vi "Deinit.vi"(8 "error in (no error)":errorcluster, 11 "AcquistionObject in":refnum<class "AcquistionObject.lvclass">) -> (0 "error out":errorcluster, 3 "AcquistionObject out":refnum<class "AcquistionObject.lvclass">)   [LabVIEW 2014, in "AcquisitionCoreObjects.lvlib" / "AcquistionObject.lvclass"]
uses:
  AcquistionObject.lvclass
  <vilib>/Utility/config.llb/NI_LVConfig.lvlib
  <vilib>/addons/database/NI_Database_API.lvlib
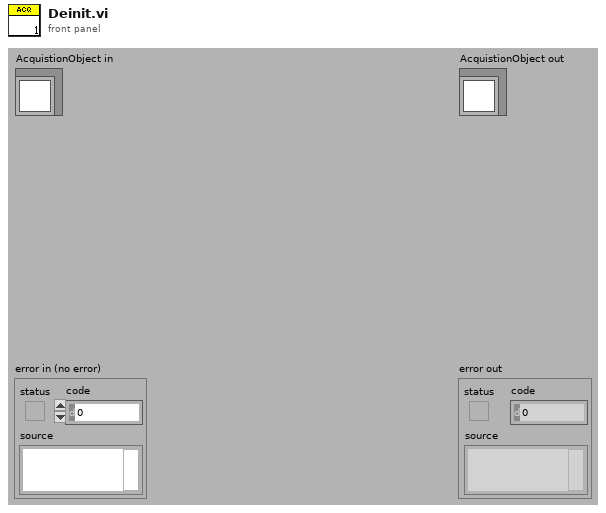
[diagram p1: front panel]
types:
  T1 = typedef "NI_Database_API.lvlib/Conn ObjectReference.ctl" = refnum<k1>
  T2 = typedef "NI_LVConfig.lvlib/Config Data RefNum.ctl" = refnum<k1>
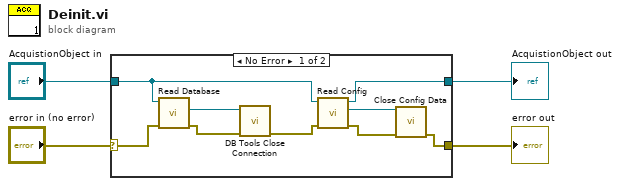
[diagram p0: block diagram]
diagram:
  n1 = case shown="No Error" "error in (no error)" {
    selector: "error in (no error)" -> [w6 w15]
    tunnel: [w5 w15] -> w3
    tunnel: [w10 w14] -> w1
    tunnel: "AcquistionObject in" -> [w11 w14]
    frame No Error {
      n2 = call-dynamic "Read Database.vi"("error in (no error)"=w6, "AcquistionObject in"=w11) -> ("error out"=w8:errorcluster, "reference"=w9:T1)  [unwired: 7 in, 1 out]
      n3 = call <vilib>:"DB Tools Close Connection.vi"("error in (no error)"=w8, "connection reference"=w9) -> ("error out"=w7:errorcluster)  [unwired: 5 in]
      n4 = call-dynamic "Read Config.vi"("error in (no error)"=w7, "AcquistionObject in"=w11) -> ("error out"=w12:errorcluster, "config data"=w13:T2, "AcquistionObject out"=w10:refnum<class "AcquistionObject.lvclass">)  [unwired: 7 in]
      n5 = call <vilib>:"Close Config Data.vi"("error in (no error)"=w12, "refnum"=w13) -> ("error out"=w5:errorcluster)  [unwired: 8 in, 1 out]
    }
    frame Error {
    }
  }
  "error out" <- w3
  "AcquistionObject out" <- w1
